vi "DMR_FindList.vi"(3 "flags IN":u32, 4 "list name IN":string, 5 "list type IN":T1(ring), 6 "driver handle IN":i32) -> (0 "error code OUT":i32, 1 "list handle OUT":i32, 2 "driver handle OUT":i32)   [LabVIEW 2014]
doc: "Locates a specified list within the device drivers interface.\n\nThis function tries to locate a certain list of device properties within the device driver interface.\n\nOnce a list has been located successfully the properties contained in that list can be accessed via the VI OBJ_GetHandle.\n\nThe 'flags IN' terminal currently is not supported for most list types However for 'HRT control' lists it serves as an index the the control machine in question.\n\nThe 'list name IN' terminal is only needed if there is more then one list of the specified type(this can e.g. be the case for setting lists).\n\nThe 'error code OUT' terminal will deliver 0 if successful or a negative error code otherwise. A list of valid error codes and their meaning can be found in the manual about this interface."
uses:
  mvDeviceManager.dll
panel:
  # "OUTPUT"
  # "INPUT"
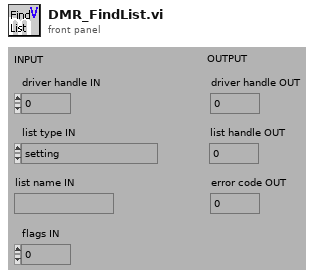
[diagram p1: front panel]
types:
  T1 = enum32{"setting", "request", "request control", "info", "statistics", "system settings", "I/O sub system", "HRT control", "camera descriptions", "device specific data", "event sub system settings", "event sub system results", "image memory manager"}
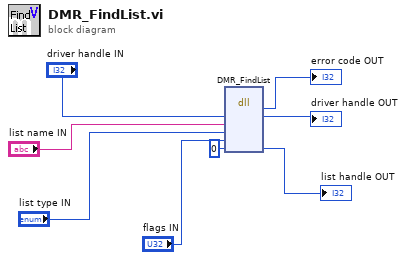
[diagram p0: block diagram]
diagram:
  n1 = dll-call lib="mvDeviceManager.dll" fn="DMR_FindList"("hDrv"="driver handle IN", "pListName"="list name IN", "listType"="list type IN", "flags"="flags IN", "pListHandle"=0) -> (→"error code OUT":i32, "hDrv"=→"driver handle OUT":i32, "pListHandle"=→"list handle OUT":i32)  [unwired: 6 in, 2 out]
